vi "Configure Clock Recovery.vi"(0 "VISA resource name":refnum<visa-resource-name>, 1 "Source (1: Channel 1)":i32(ring) items=["Channel 1", "Channel 2", "Channel 3", "Channel 4", "Function 1", "Function 2", "Function 3", "Function 4", "Memory 1", "Memory 2", "Memory 3", "Memory 4"], 2 "Clock Recovery Method (4: Constant Frequency)":i32(ring) items=["PCI Express", "Fibre Channel", "First Order PLL", "Second Order PLL", "Constant Frequency", "Explicit Clock", "Explicit First Order PLL", "Explicit Second Order PLL"], 3 "Nominal Data Rate (2.5E9 Hz)":dbl, 4 "Loop Bandwidth (1.4997E6 Hz)":dbl, 5 "Clock Edge (0: Rising)":i32(ring) items=["Rising", "Falling", "Both"], 6 "Clock Frequency (2.5E9 Hz)":dbl, 7 "error in (no error)":errorcluster, 8 "Enable Recovered Clock Display (Enable)":bool, 9 "Data Rate Type (0: Fully Automatic)":i32(ring) items=["Fully Automatic", "Semi-Automatic", "Manual"], 11 "Fibre Channel (0: FC1063)":i32(ring) items=["FC1063", "FC2125", "FC425"], 13 "Clock Multiplier (1)":u32, 15 "Damping Factor (1 bits/s)":dbl format="%#.3g", 17 "Data Bits (0: Both)":i32(ring) items=["Both", "Deemphasis", "Transition"], 19 "Vertical":T1 {"Vertical Scale Mode (0: Automatic)" items=["Automatic", "Manual"]}) -> (20 "VISA resource name out":refnum<visa-resource-name>, 27 "error out":errorcluster)   [LabVIEW 2009, in "Agilent 8000 Series.lvlib"]
doc: "Configures the Clock Recovery Parameters."
uses:
  Agilent 8000 Series.lvlib
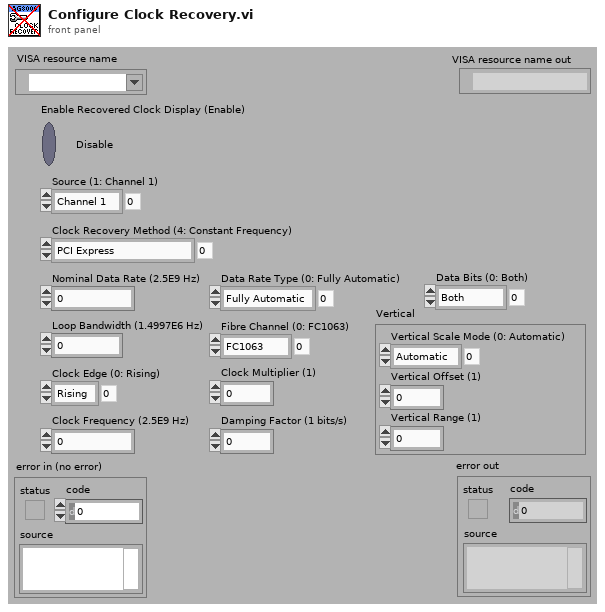
[diagram p1: front panel]
types:
  T1 = cluster{"Vertical Range (1)":dbl, "Vertical Offset (1)":dbl, "Vertical Scale Mode (0: Automatic)":i32}
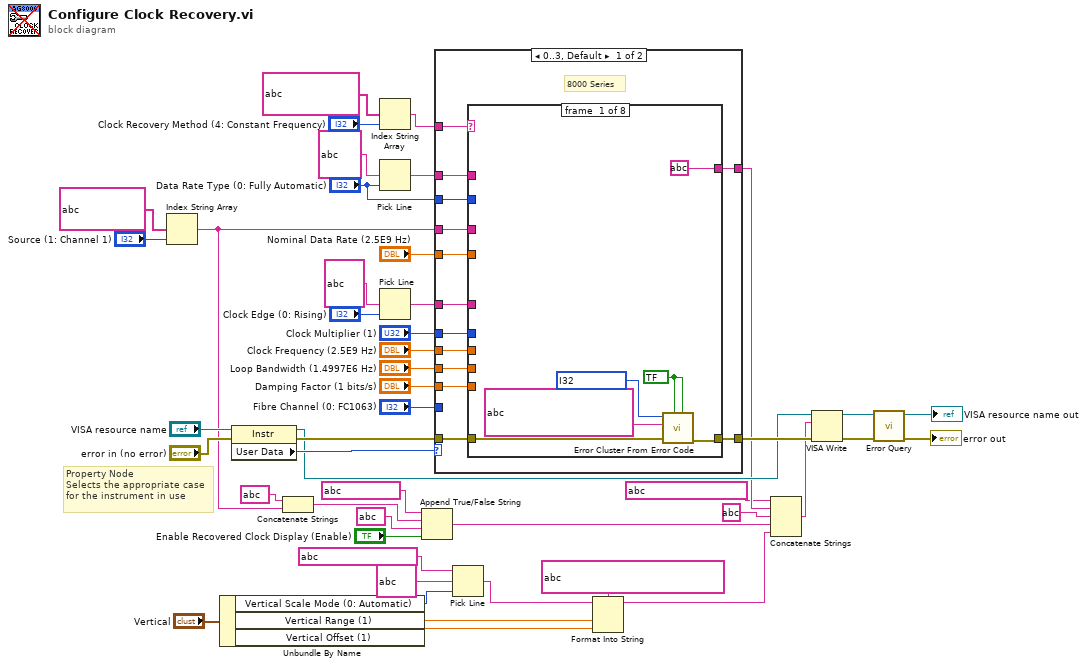
[diagram p0: block diagram]
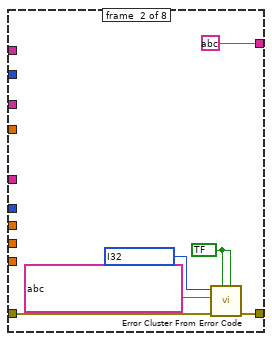
[diagram p2: hidden frame]
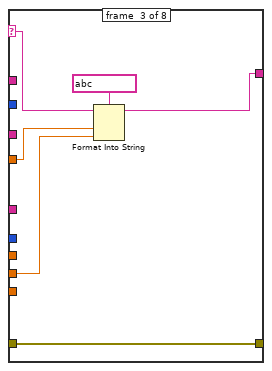
[diagram p3: hidden frame]
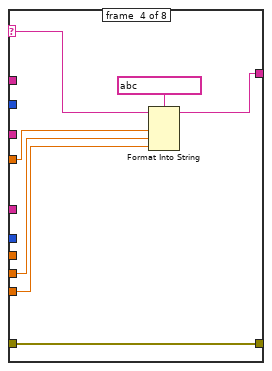
[diagram p4: hidden frame]
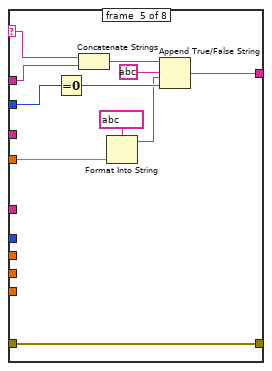
[diagram p5: hidden frame]
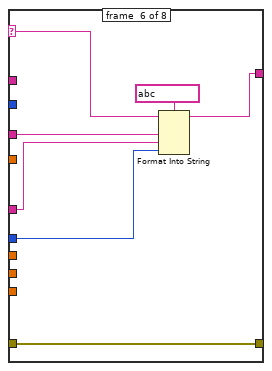
[diagram p6: hidden frame]
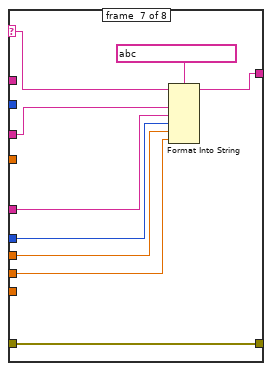
[diagram p7: hidden frame]
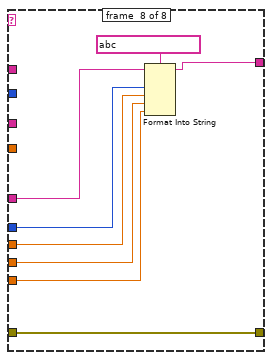
[diagram p8: hidden frame]
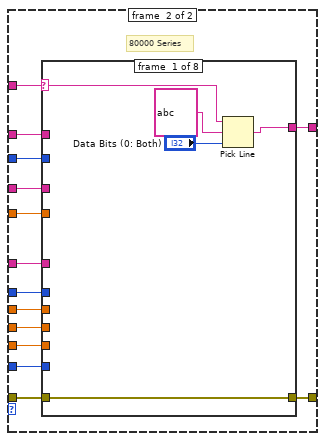
[diagram p9: hidden frame]
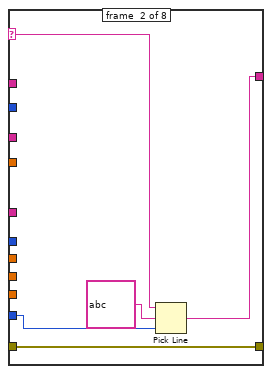
[diagram p10: hidden frame]
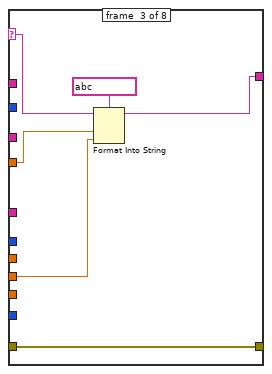
[diagram p11: hidden frame]
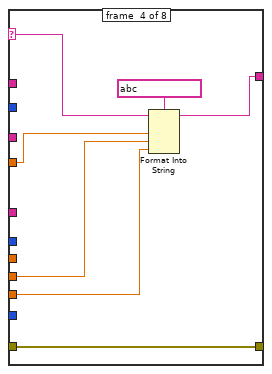
[diagram p12: hidden frame]
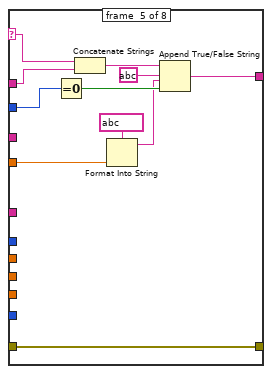
[diagram p13: hidden frame]
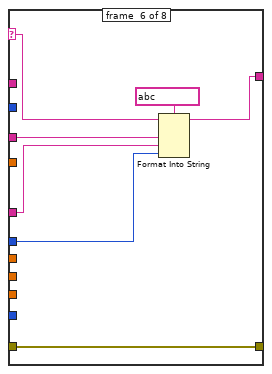
[diagram p14: hidden frame]
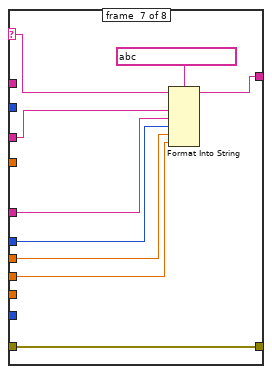
[diagram p15: hidden frame]
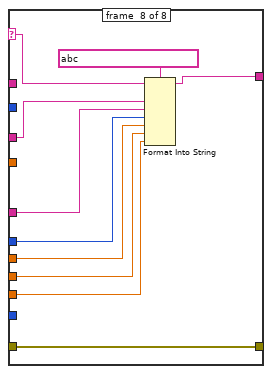
[diagram p16: hidden frame]
diagram:
  # "Property Node\nSelects the appropriate case\nfor the instrument in use"
  n1 = Index String Array(1:"Source (1: Channel 1)", 2:string[] ?) -> (0:w12:string)  [unwired: 1 in]
  n2 = Unbundle By Name("Vertical") -> ("Vertical Scale Mode (0: Automatic)"=w18:i32, "Vertical Range (1)"=w21:dbl, "Vertical Offset (1)"=w20:dbl)
  n3 = property class="Instr"(reference="VISA resource name", error in="error in (no error)") -> (reference out=w22:refnum<visa-resource-name>, error out=w24:errorcluster, "User Data"=w26:u32)
  n4 = Concatenate Strings(string ? ("string"), w12) -> (w10:string)
  n5 = Index String Array(1:"Clock Recovery Method (4: Constant Frequency)", 2:string[] ?) -> (0:w28:string)  [unwired: 1 in]
  n6 = Pick Line(multi-line string=string ?, line index="Data Rate Type (0: Fully Automatic)") -> (output string=w29:string)  [unwired: 1 in]
  n7 = Pick Line(multi-line string=string ?, line index="Clock Edge (0: Rising)") -> (output string=w31:string)  [unwired: 1 in]
  n8 = Append True/False String(1:"Enable Recovered Clock Display (Enable)", 2:string ? ("string"), 3:w10, 4:string ? ("string (\"\")")) -> (0:w7:string)
  n9 = case shown="0..3, Default" w26 {
    tunnel: "Loop Bandwidth (1.4997E6 Hz)" -> [w60 w134]
    tunnel: "Nominal Data Rate (2.5E9 Hz)" -> [w59 w133]
    tunnel: "Damping Factor (1 bits/s)" -> [w58 w132]
    tunnel: "Clock Multiplier (1)" -> [w57 w131]
    tunnel: "Clock Frequency (2.5E9 Hz)" -> [w56 w130]
    tunnel: w12 -> [w55 w129]
    tunnel: w31 -> [w54 w128]
    tunnel: w29 -> [w53 w127]
    tunnel: w28 -> [w52 w126]
    tunnel: "Data Rate Type (0: Fully Automatic)" -> [w51 w125]
    tunnel: "Fibre Channel (0: FC1063)" -> [_ w124]
    tunnel: [w50 w123] -> w3
    tunnel: w24 -> [w49 w122]
    tunnel: [w48 w121] -> w23
    frame #0 {
      # "8000 Series"
      n10 = case shown="\"FIX\", Default" w52 {
        selector: w52 -> [_ _ w75 w84 w88 w101 w108 _]
        tunnel: w59 -> [_ _ w78 w83 w96 _ _ _]
        tunnel: w60 -> [_ _ w77 w82 _ _ w110 w117]
        tunnel: w58 -> [_ _ _ w81 _ _ _ w116]
        tunnel: w57 -> [_ _ _ _ _ w100 w109 w118]
        tunnel: w56 -> [_ _ _ _ _ _ w111 w119]
        tunnel: w55 -> [_ _ _ _ _ w102 w107 _]
        tunnel: w54 -> [_ _ _ _ _ w99 w106 w115]
        tunnel: w53 -> [_ _ _ _ w87 _ _ _]
        tunnel: w51 -> [_ _ _ _ w94 _ _ _]
        tunnel: [string ? string ? w74 w80 w89 w98 w105 w114] -> w50
        tunnel: w49 -> [w63 w69 w73 w79 w90 w97 w104 w113]
        tunnel: [w62 w68 w73 w79 w90 w97 w104 w113] -> w48
        frame #0 {
          w64 = bool ? ("is warning? (False)")
          n11 = call <vilib>:"Error Cluster From Error Code.vi"("is warning? (False)"=w64, "show call chain? (False)"=w64, "error in (no error)"=w63, "error message (\"\")"=string ? ("error message (\"\")"), "error code (0)"=i32 ? ("Code")) -> ("error out"=w62:errorcluster)  [unwired: 4 in]
        }
        frame #1 {
          w70 = bool ? ("is warning? (False)")
          n12 = call <vilib>:"Error Cluster From Error Code.vi"("is warning? (False)"=w70, "show call chain? (False)"=w70, "error in (no error)"=w69, "error message (\"\")"=string ? ("error message (\"\")"), "error code (0)"=i32 ? ("Code")) -> ("error out"=w68:errorcluster)  [unwired: 4 in]
        }
        frame #2 {
          n13 = Format Into String(format string=string ?, initial string=w75, w78, w77) -> (resulting string=w74:string)  [unwired: 1 in, 1 out]
        }
        frame #3 {
          n14 = Format Into String(format string=string ?, initial string=w84, w83, w82, w81) -> (resulting string=w80:string)  [unwired: 1 in, 1 out]
        }
        frame #4 {
          n15 = Equal To 0?(x=w94) -> (x = 0?=w93:bool)
          n16 = Concatenate Strings(w88, w87) -> (w86:string)
          n17 = Format Into String(format string=string ?, w96) -> (resulting string=w91:string)  [unwired: 2 in, 1 out]
          n18 = Append True/False String(1:w93, 2:w91, 3:string ?, 4:w86) -> (0:w89:string)
        }
        frame #5 {
          n19 = Format Into String(format string=string ?, initial string=w101, w102, w99, w100) -> (resulting string=w98:string)  [unwired: 1 in, 1 out]
        }
        frame #6 {
          n20 = Format Into String(format string=string ?, initial string=w108, w107, w106, w109, w111, w110) -> (resulting string=w105:string)  [unwired: 1 in, 1 out]
        }
        frame #7 {
          n21 = Format Into String(format string=string ?, initial string=w115, w118, w119, w117, w116) -> (resulting string=w114:string)  [unwired: 1 in, 1 out]
        }
      }
    }
    frame #1 {
      # "80000 Series"
      n22 = case shown="\"FIX\", Default" w126 {
        selector: w126 -> [w137 w142 w147 w156 w160 w173 w180 w185]
        tunnel: w133 -> [_ _ w150 w155 w168 _ _ _]
        tunnel: w134 -> [_ _ w149 w154 _ _ w182 w192]
        tunnel: w132 -> [_ _ _ w153 _ _ _ w191]
        tunnel: w131 -> [_ _ _ _ _ w172 w181 w188]
        tunnel: w130 -> [_ _ _ _ _ _ w183 w193]
        tunnel: w129 -> [_ _ _ _ _ w174 w179 w186]
        tunnel: w128 -> [_ _ _ _ _ w171 w178 w187]
        tunnel: w127 -> [_ _ _ _ w159 _ _ _]
        tunnel: w125 -> [_ _ _ _ w166 _ _ _]
        tunnel: [w136 w141 w146 w152 w161 w170 w177 w190] -> w123
        tunnel: w124 -> [_ w144 _ _ _ _ _ _]
        tunnel: w122 -> [w139 w140 w145 w151 w162 w169 w176 w189]
        tunnel: [w139 w140 w145 w151 w162 w169 w176 w189] -> w121
        frame #0 {
          n23 = Pick Line(string ("")=w137, multi-line string=string ?, line index="Data Bits (0: Both)") -> (output string=w136:string)
        }
        frame #1 {
          n24 = Pick Line(string ("")=w142, multi-line string=string ?, line index=w144) -> (output string=w141:string)
        }
        frame #2 {
          n25 = Format Into String(format string=string ?, initial string=w147, w150, w149) -> (resulting string=w146:string)  [unwired: 1 in, 1 out]
        }
        frame #3 {
          n26 = Format Into String(format string=string ?, initial string=w156, w155, w154, w153) -> (resulting string=w152:string)  [unwired: 1 in, 1 out]
        }
        frame #4 {
          n27 = Equal To 0?(x=w166) -> (x = 0?=w165:bool)
          n28 = Concatenate Strings(w160, w159) -> (w158:string)
          n29 = Format Into String(format string=string ?, w168) -> (resulting string=w163:string)  [unwired: 2 in, 1 out]
          n30 = Append True/False String(1:w165, 2:w163, 3:string ?, 4:w158) -> (0:w161:string)
        }
        frame #5 {
          n31 = Format Into String(format string=string ?, initial string=w173, w174, w171, w172) -> (resulting string=w170:string)  [unwired: 1 in, 1 out]
        }
        frame #6 {
          n32 = Format Into String(format string=string ?, initial string=w180, w179, w178, w181, w183, w182) -> (resulting string=w177:string)  [unwired: 1 in, 1 out]
        }
        frame #7 {
          n33 = Format Into String(format string=string ?, initial string=w185, w186, w187, w188, w193, w192, w191) -> (resulting string=w190:string)  [unwired: 1 in, 1 out]
        }
      }
    }
  }
  n34 = Pick Line(string ("")=string ?, multi-line string=string ?, line index=w18) -> (output string=w17:string)
  n35 = Format Into String(format string=string ?, initial string=w17, w21, w20) -> (resulting string=w6:string)  [unwired: 1 in, 1 out]
  n36 = Concatenate Strings(string ? ("format string"), w3, string ? ("string"), w7, w6) -> (w5:string)
  n37 = VISA Write(VISA resource name=w22, write buffer=w5, error in (no error)=w23) -> (VISA resource name out=w43:refnum<visa-resource-name>, error out=w42:errorcluster)  [unwired: 1 out]
  n38 = call "Error Query.vi"("error in (no error)"=w42, "VISA resource name"=w43) -> ("error out"=→"error out":errorcluster, "VISA resource name out"=→"VISA resource name out":refnum<visa-resource-name>)  [unwired: 6 in, 2 out]
